vi "user_new.vi"(8 "error in (no error)":errorcluster) -> (0 "error IO":errorcluster, 1 "cancelled?":bool, 2 "user name out":string)   [LabVIEW 2010]
panel:
  in  "cancel":bool
  in  "save":bool
  in  "user name":string caption="new user name:"
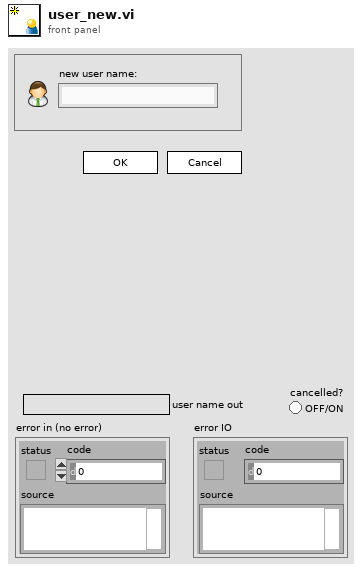
[diagram p1: front panel]
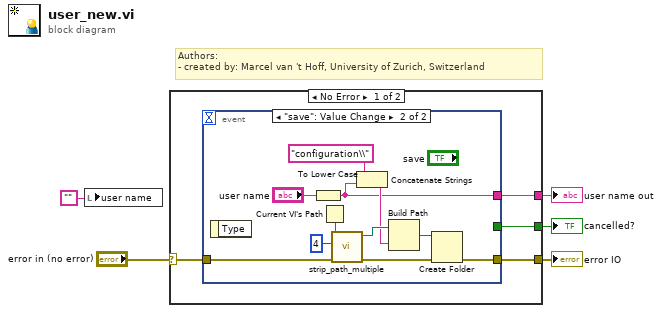
[diagram p0: block diagram]
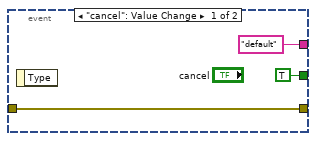
[diagram p2: hidden frame]
diagram:
  # "Authors: \n- created by: Marcel van 't Hoff, University of Zurich, Switzerland"
  n1 = local write "user name"("") -> ()
  n2 = case shown="No Error" "error in (no error)" {
    selector: "error in (no error)" -> [w9 w24]
    tunnel: [w8 w24] -> w4
    tunnel: [w7 _] -> w3
    tunnel: [w6 _] -> w1
    frame No Error {
      n3 = event shown="[1] \"save\": Value Change" {
        selector: _ -> [_ _]
        dyn-events: _ -> [_ _]
        timeout: _ -> [_ _]
        tunnel: w9 -> [w12 w23]
        tunnel: [w12 w15] -> w8
        tunnel: ["default" ("user name") w13] -> w7
        tunnel: [TRUE ("cancel") _] -> w6
        event "cancel": Value Change {
          n4 = event-data() -> ()  [unwired: 1 in, 1 out]
        }
        event "save": Value Change {
          n5 = event-data() -> ()  [unwired: 1 in, 1 out]
          n6 = To Lower Case(string="user name") -> (all lower case string=w13:string)
          n7 = Current VI's Path() -> (path=w22:path)
          n8 = call "strip_path_multiple.vi"("error in (no error)"=w23, "number of strips"=4, "path in"=w22) -> ("error out"=w16:errorcluster, "path out"=w20:path)  [unwired: 7 in]
          n9 = Concatenate Strings("configuration\\" ("name or relative path"), w13) -> (w18:string)
          n10 = Build Path(base path=w20, name or relative path=w18) -> (appended path=w17:path)
          n11 = Create Folder(path (use dialog)=w17, error in=w16) -> (error out=w15:errorcluster)  [unwired: 1 in, 2 out]
        }
      }
    }
    frame Error {
    }
  }
  "error IO" <- w4
  "user name out" <- w3
  "cancelled?" <- w1
